vi "Wrap Angle (scalar).vi"(7 "angle units":T2 items=["radian in, radian out", "radian in, degree out", "degree in, degree out", "degree in, radian out"], 10 "angle range":T1=1 items=["none", "-180 to 180 (-pi to pi)", "0 to 360 (0 to 2pi)"], 11 "angle in":dbl) -> (0 "error":i32, 3 "angle out":dbl)   [LabVIEW 2017, in "NI_AAL_Angle.lvlib"]
doc: "Wraps the input angle to a value within the range you specify with <B>angle range</B>.\n\nWire data to any of the angle inputs to determine the polymorphic instance to use or manually select the instance."
uses:
  <vilib>/Analysis/NI_AAL_Angle.lvlib
  <vilib>/Analysis/coordinate.llb/Angle Units.ctl
  <vilib>/Analysis/coordinate.llb/Angle Range (Degree).ctl
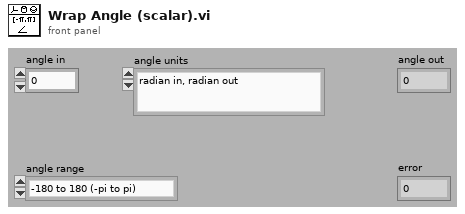
[diagram p1: front panel]
types:
  T1 = typedef "NI_AAL_Angle.lvlib/Angle Range (Degree).ctl" = u16
  T2 = typedef "NI_AAL_Angle.lvlib/Angle Units.ctl" = i32
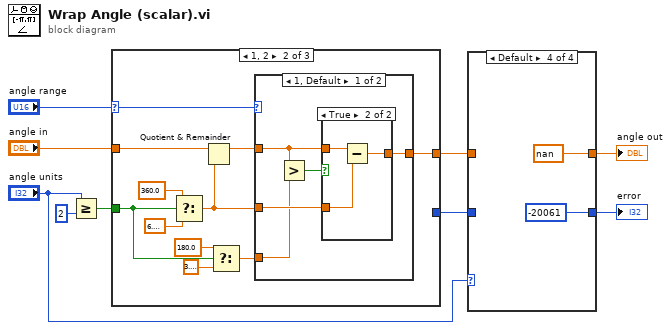
[diagram p0: block diagram]
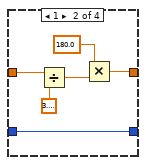
[diagram p3: hidden frame]
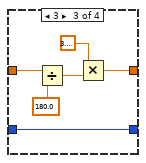
[diagram p4: hidden frame]
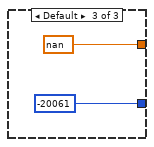
[diagram p8: hidden frame]
diagram:
  n1 = Greater Or Equal?(x="angle units", y=2) -> (x >= y?=w7:bool)
  n2 = case shown="1, 2" "angle range" {
    selector: "angle range" -> [_ w18 _]
    tunnel: "angle in" -> [w10 w20 _]
    tunnel: [w10 w19 nan ("angle in")] -> w6
    tunnel: [_ _ -20061] -> w5
    tunnel: w7 -> [_ w14 _]
    frame 0 {
    }
    frame 1, 2 {
      n3 = Select(t=360.0, s=w14, f=6.283185307179586) -> (s? t:f=w15:dbl)
      n4 = Quotient & Remainder(x=w20, y=w15) -> (x-y*floor(x/y)=w21:dbl)  [unwired: 1 out]
      n5 = Select(t=180.0, s=w14, f=3.141592653589793) -> (s? t:f=w11:dbl)
      n6 = case shown="1, Default" w18 {
        tunnel: w21 -> [w26 w31]
        tunnel: [w24 w31] -> w19
        tunnel: w15 -> [w23 _]
        tunnel: w11 -> [w22 _]
        frame 1, Default {
          n7 = Greater?(x=w26, y=w22) -> (0:w25:bool)
          n8 = case shown="True" w25 {
            tunnel: w26 -> [w27 w30]
            tunnel: [w27 w29] -> w24
            tunnel: w23 -> [_ w28]
            frame False {
            }
            frame True {
              n9 = Subtract(x=w30, y=w28) -> (x-y=w29:dbl)
            }
          }
        }
        frame 2 {
        }
      }
    }
    frame Default {
    }
  }
  n10 = case shown="Default" "angle units" {
    tunnel: w6 -> [w34 w40 w45 _]
    tunnel: w5 -> [w35 w41 w47 _]
    tunnel: [w35 w41 w47 -20061] -> w3
    tunnel: [w34 w38 w44 nan ("angle in")] -> w2
    frame 0, 2 {
    }
    frame 1 {
      n11 = Divide(x=w40, y=3.141592653589793) -> (x/y=w37:dbl)
      n12 = Multiply(x=180.0, y=w37) -> (x*y=w38:dbl)
    }
    frame 3 {
      n13 = Divide(x=w45, y=180.0 ("x")) -> (x/y=w46:dbl)
      n14 = Multiply(x=3.141592653589793, y=w46) -> (x*y=w44:dbl)
    }
    frame Default {
    }
  }
  "angle out" <- w2
  "error" <- w3
